vi "Convert CMYK to RGB.vi"(8 "K (%)":dbl format="%#_2p", 9 "Y (%)":dbl, 10 "M (%)":dbl, 11 "C (%)":dbl) -> (3 "Color out":u32(colorbox)=16777215)   [LabVIEW 2015, in "ColorSelector.lvclass"]
doc: "This VI will convert the CMYK Color Scale to the RGB Color Scale.\n<b> </b> <b> </b>\n©2017 Q Software Innovations, LLC (QSI)\nwritten by Quentin Alldredge\nproduced in LabVIEW 2015\n\nsupport@qsoftwareinnovations.com\nwww.qsoftwareinnovations.com\n\nAll rights reserved.\n\nRedistribution and use in source and binary forms, with or without modification, are permitted provided that the following conditions are met:\n\n * Redistributions of source code must retain the above copyright notice, this list of conditions and the following disclaimer.\n * Redistributions in binary form must reproduce the above copyright notice, this list of conditions and the following disclaimer in the documentation and/or other materials provided with the distribution.\n * Neither the name of Q Software Innovations, LLC. nor the names of its contributors may be used to endorse or promote products derived from this software without specific prior written permission.\n\nTHIS SOFTWARE IS PROVIDED BY THE COPYRIGHT HOLDERS AND CONTRIBUTORS \"AS IS\" AND ANY EXPRESS OR IMPLIED WARRANTIES, INCLUDING, BUT NOT LIMITED TO, THE IMPLIED WARRANTIES OF MERCHANTABILITY AND FITNESS FOR A PARTICULAR PURPOSE ARE DISCLAIMED. IN NO EVENT SHALL THE COPYRIGHT OWNER OR CONTRIBUTORS BE LIABLE FOR ANY DIRECT, INDIRECT, INCIDENTAL, SPECIAL, EXEMPLARY, OR CONSEQUENTIAL DAMAGES (INCLUDING, BUT NOT LIMITED TO, PROCUREMENT OF SUBSTITUTE GOODS OR SERVICES; LOSS OF USE, DATA, OR PROFITS; OR BUSINESS INTERRUPTION) HOWEVER CAUSED AND ON ANY THEORY OF LIABILITY, WHETHER IN CONTRACT, STRICT LIABILITY, OR TORT (INCLUDING NEGLIGENCE OR OTHERWISE) ARISING IN ANY WAY OUT OF THE USE OF THIS SOFTWARE, EVEN IF ADVISED OF THE POSSIBILITY OF SUCH DAMAGE."
uses:
  ColorSelector.lvclass
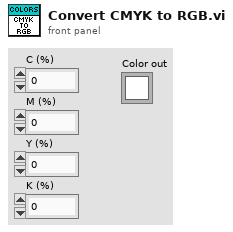
[diagram p1: front panel]
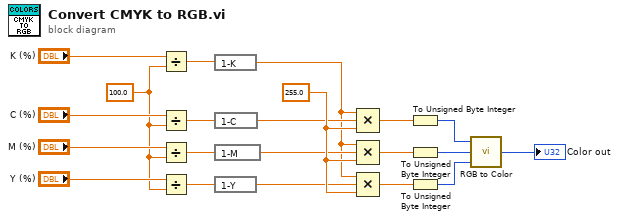
[diagram p0: block diagram]
diagram:
  w14 = 255.0 ("y")
  w1 = 100.0 ("y")
  n1 = Divide(x="K (%)", y=w1) -> (x/y=w10:dbl)
  n2 = Divide(x="C (%)", y=w1) -> (x/y=w17:dbl)
  n3 = Divide(x="M (%)", y=w1) -> (x/y=w16:dbl)
  n4 = Divide(x="Y (%)", y=w1) -> (x/y=w15:dbl)
  n5 = expression code="1-K"(w10) -> (w9:dbl)
  n6 = expression code="1-C"(w17) -> (w13:dbl)
  n7 = expression code="1-M"(w16) -> (w12:dbl)
  n8 = expression code="1-Y"(w15) -> (w11:dbl)
  n9 = Compound Arithmetic op=MULTIPLY(w9, w13, w14) -> (w8:dbl)
  n10 = Compound Arithmetic op=MULTIPLY(w9, w12, w14) -> (w7:dbl)
  n11 = Compound Arithmetic op=MULTIPLY(w9, w11, w14) -> (w6:dbl)
  n12 = To Unsigned Byte Integer(number=w8) -> (unsigned 8bit integer=w4:u8)
  n13 = To Unsigned Byte Integer(number=w7) -> (unsigned 8bit integer=w5:u8)
  n14 = To Unsigned Byte Integer(number=w6) -> (unsigned 8bit integer=w3:u8)
  n15 = call <vilib>:"RGB to Color.vi"("B"=w3, "G"=w5, "R"=w4) -> ("Color"=→"Color out":u32)
